vi "Experiment 6.vi"() -> ()   [LabVIEW 2026]
doc: "Experiment 6"
uses:
  <vilib>/Analysis/baseanly.llb/Mean (DBL).vi
  <vilib>/Analysis/NI_AALBase.lvlib
panel:
  out "Execution Time - Per Call (us)":dbl format="%.6f"
  out "Execution Time - 1M Calls (seconds)":dbl format="%.6f"
  out "Output":dbl[](array[numeric]) format="%.3f"
  # "Experiment 6"
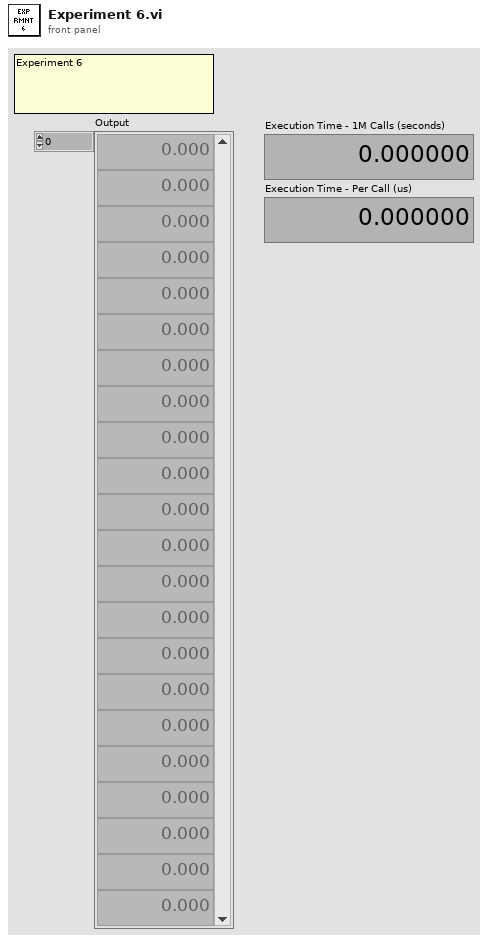
[diagram p1: front panel]
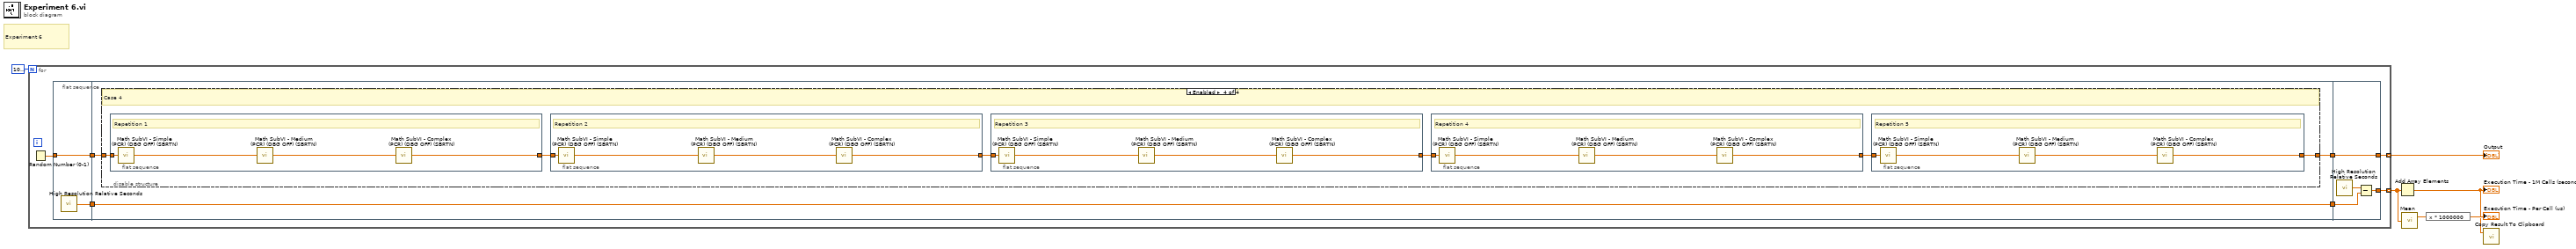
[diagram p0: block diagram]
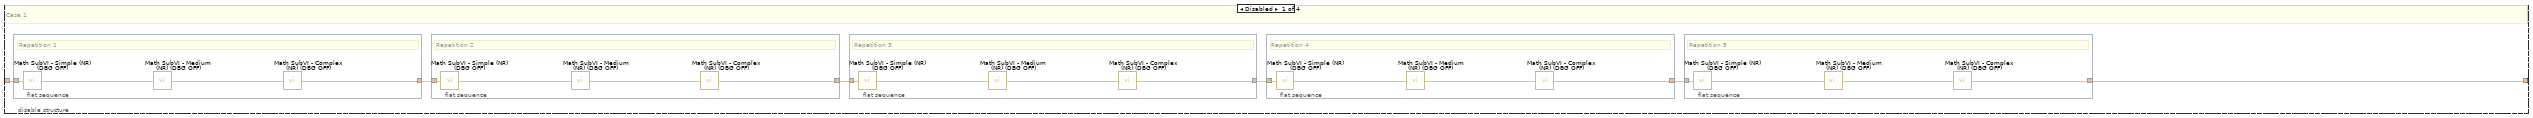
[diagram p2: hidden frame]
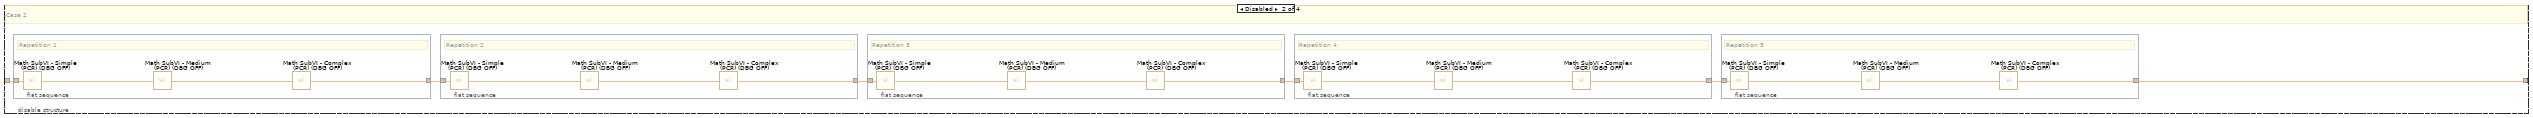
[diagram p3: hidden frame]
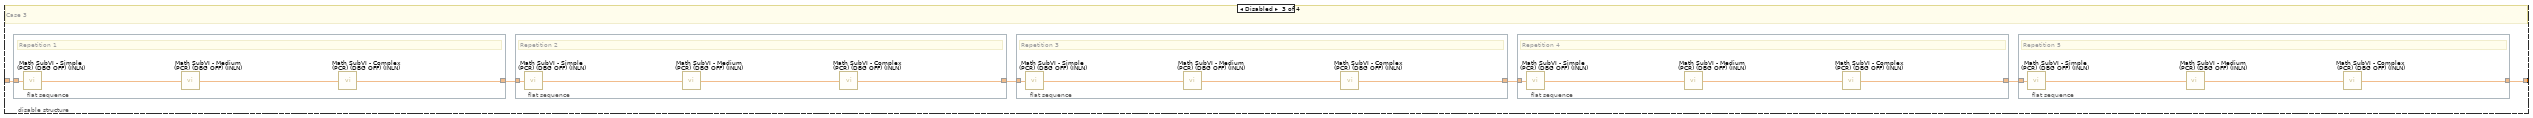
[diagram p4: hidden frame]
diagram:
  # "Experiment 6"
  n1 = for {
    N: 1000000 -> [_]
    tunnel: [w13] -> w6 mode=indexing
    tunnel: [w7] -> w4 mode=indexing
    n2 = Random Number (0-1)() -> (number: 0 to 1=w12:dbl)
    n3 = flat-sequence {
      tunnel: w12 -> [w15]
      tunnel: [w15] -> w11
      tunnel: [w14] -> w8
      tunnel: w11 -> [w16]
      tunnel: [w17] -> w10
      tunnel: [w18] -> w9
      tunnel: w8 -> [w18]
      tunnel: [w126] -> w13
      tunnel: w10 -> [w126]
      tunnel: w9 -> [w124]
      tunnel: [w123] -> w7
      frame #0 {
        n4 = call <vilib>:"High Resolution Relative Seconds.vi"() -> ("relative seconds"=w14:dbl)
      }
      frame #1 {
        n5 = disable-structure shown="Enabled" {
          disable-tunnel: [w19 w45 w71 w97] -> w17
          disable-tunnel: w16 -> [w24 w50 w76 w102]
          frame Disabled {
            # "Case 1"
            n6 = flat-sequence {
              tunnel: w24 -> [w43]
              tunnel: [w41] -> w23
              frame #0 {
                # "Repetition 1"
                n7 = call "Math SubVI - Simple (NR) (DBG OFF).vi"("Input"=w43) -> ("Output"=w44:dbl)
                n8 = call "Math SubVI - Medium (NR) (DBG OFF).vi"("Input"=w44) -> ("Output"=w42:dbl)
                n9 = call "Math SubVI - Complex (NR) (DBG OFF).vi"("Input"=w42) -> ("Output"=w41:dbl)
              }
            }
            n10 = flat-sequence {
              tunnel: w23 -> [w39]
              tunnel: [w37] -> w22
              frame #0 {
                # "Repetition 2"
                n11 = call "Math SubVI - Simple (NR) (DBG OFF).vi"("Input"=w39) -> ("Output"=w40:dbl)
                n12 = call "Math SubVI - Medium (NR) (DBG OFF).vi"("Input"=w40) -> ("Output"=w38:dbl)
                n13 = call "Math SubVI - Complex (NR) (DBG OFF).vi"("Input"=w38) -> ("Output"=w37:dbl)
              }
            }
            n14 = flat-sequence {
              tunnel: w22 -> [w35]
              tunnel: [w33] -> w21
              frame #0 {
                # "Repetition 3"
                n15 = call "Math SubVI - Simple (NR) (DBG OFF).vi"("Input"=w35) -> ("Output"=w36:dbl)
                n16 = call "Math SubVI - Medium (NR) (DBG OFF).vi"("Input"=w36) -> ("Output"=w34:dbl)
                n17 = call "Math SubVI - Complex (NR) (DBG OFF).vi"("Input"=w34) -> ("Output"=w33:dbl)
              }
            }
            n18 = flat-sequence {
              tunnel: w21 -> [w31]
              tunnel: [w29] -> w20
              frame #0 {
                # "Repetition 4"
                n19 = call "Math SubVI - Simple (NR) (DBG OFF).vi"("Input"=w31) -> ("Output"=w32:dbl)
                n20 = call "Math SubVI - Medium (NR) (DBG OFF).vi"("Input"=w32) -> ("Output"=w30:dbl)
                n21 = call "Math SubVI - Complex (NR) (DBG OFF).vi"("Input"=w30) -> ("Output"=w29:dbl)
              }
            }
            n22 = flat-sequence {
              tunnel: w20 -> [w27]
              tunnel: [w25] -> w19
              frame #0 {
                # "Repetition 5"
                n23 = call "Math SubVI - Simple (NR) (DBG OFF).vi"("Input"=w27) -> ("Output"=w28:dbl)
                n24 = call "Math SubVI - Medium (NR) (DBG OFF).vi"("Input"=w28) -> ("Output"=w26:dbl)
                n25 = call "Math SubVI - Complex (NR) (DBG OFF).vi"("Input"=w26) -> ("Output"=w25:dbl)
              }
            }
          }
          frame Disabled {
            # "Case 2"
            n26 = flat-sequence {
              tunnel: w50 -> [w69]
              tunnel: [w67] -> w49
              frame #0 {
                # "Repetition 1"
                n27 = call "Math SubVI - Simple (PCR) (DBG OFF).vi"("Input"=w69) -> ("Output"=w70:dbl)
                n28 = call "Math SubVI - Medium (PCR) (DBG OFF).vi"("Input"=w70) -> ("Output"=w68:dbl)
                n29 = call "Math SubVI - Complex (PCR) (DBG OFF).vi"("Input"=w68) -> ("Output"=w67:dbl)
              }
            }
            n30 = flat-sequence {
              tunnel: w49 -> [w65]
              tunnel: [w63] -> w48
              frame #0 {
                # "Repetition 2"
                n31 = call "Math SubVI - Simple (PCR) (DBG OFF).vi"("Input"=w65) -> ("Output"=w66:dbl)
                n32 = call "Math SubVI - Medium (PCR) (DBG OFF).vi"("Input"=w66) -> ("Output"=w64:dbl)
                n33 = call "Math SubVI - Complex (PCR) (DBG OFF).vi"("Input"=w64) -> ("Output"=w63:dbl)
              }
            }
            n34 = flat-sequence {
              tunnel: w48 -> [w61]
              tunnel: [w59] -> w47
              frame #0 {
                # "Repetition 3"
                n35 = call "Math SubVI - Simple (PCR) (DBG OFF).vi"("Input"=w61) -> ("Output"=w62:dbl)
                n36 = call "Math SubVI - Medium (PCR) (DBG OFF).vi"("Input"=w62) -> ("Output"=w60:dbl)
                n37 = call "Math SubVI - Complex (PCR) (DBG OFF).vi"("Input"=w60) -> ("Output"=w59:dbl)
              }
            }
            n38 = flat-sequence {
              tunnel: w47 -> [w57]
              tunnel: [w55] -> w46
              frame #0 {
                # "Repetition 4"
                n39 = call "Math SubVI - Simple (PCR) (DBG OFF).vi"("Input"=w57) -> ("Output"=w58:dbl)
                n40 = call "Math SubVI - Medium (PCR) (DBG OFF).vi"("Input"=w58) -> ("Output"=w56:dbl)
                n41 = call "Math SubVI - Complex (PCR) (DBG OFF).vi"("Input"=w56) -> ("Output"=w55:dbl)
              }
            }
            n42 = flat-sequence {
              tunnel: w46 -> [w53]
              tunnel: [w51] -> w45
              frame #0 {
                # "Repetition 5"
                n43 = call "Math SubVI - Simple (PCR) (DBG OFF).vi"("Input"=w53) -> ("Output"=w54:dbl)
                n44 = call "Math SubVI - Medium (PCR) (DBG OFF).vi"("Input"=w54) -> ("Output"=w52:dbl)
                n45 = call "Math SubVI - Complex (PCR) (DBG OFF).vi"("Input"=w52) -> ("Output"=w51:dbl)
              }
            }
          }
          frame Disabled {
            # "Case 3"
            n46 = flat-sequence {
              tunnel: w76 -> [w95]
              tunnel: [w93] -> w75
              frame #0 {
                # "Repetition 1"
                n47 = call "Math SubVI - Simple (PCR) (DBG OFF) (INLN).vi"("Input"=w95) -> ("Output"=w96:dbl)
                n48 = call "Math SubVI - Medium (PCR) (DBG OFF) (INLN).vi"("Input"=w96) -> ("Output"=w94:dbl)
                n49 = call "Math SubVI - Complex (PCR) (DBG OFF) (INLN).vi"("Input"=w94) -> ("Output"=w93:dbl)
              }
            }
            n50 = flat-sequence {
              tunnel: w75 -> [w91]
              tunnel: [w89] -> w74
              frame #0 {
                # "Repetition 2"
                n51 = call "Math SubVI - Simple (PCR) (DBG OFF) (INLN).vi"("Input"=w91) -> ("Output"=w92:dbl)
                n52 = call "Math SubVI - Medium (PCR) (DBG OFF) (INLN).vi"("Input"=w92) -> ("Output"=w90:dbl)
                n53 = call "Math SubVI - Complex (PCR) (DBG OFF) (INLN).vi"("Input"=w90) -> ("Output"=w89:dbl)
              }
            }
            n54 = flat-sequence {
              tunnel: w74 -> [w87]
              tunnel: [w85] -> w73
              frame #0 {
                # "Repetition 3"
                n55 = call "Math SubVI - Simple (PCR) (DBG OFF) (INLN).vi"("Input"=w87) -> ("Output"=w88:dbl)
                n56 = call "Math SubVI - Medium (PCR) (DBG OFF) (INLN).vi"("Input"=w88) -> ("Output"=w86:dbl)
                n57 = call "Math SubVI - Complex (PCR) (DBG OFF) (INLN).vi"("Input"=w86) -> ("Output"=w85:dbl)
              }
            }
            n58 = flat-sequence {
              tunnel: w73 -> [w83]
              tunnel: [w81] -> w72
              frame #0 {
                # "Repetition 4"
                n59 = call "Math SubVI - Simple (PCR) (DBG OFF) (INLN).vi"("Input"=w83) -> ("Output"=w84:dbl)
                n60 = call "Math SubVI - Medium (PCR) (DBG OFF) (INLN).vi"("Input"=w84) -> ("Output"=w82:dbl)
                n61 = call "Math SubVI - Complex (PCR) (DBG OFF) (INLN).vi"("Input"=w82) -> ("Output"=w81:dbl)
              }
            }
            n62 = flat-sequence {
              tunnel: w72 -> [w79]
              tunnel: [w77] -> w71
              frame #0 {
                # "Repetition 5"
                n63 = call "Math SubVI - Simple (PCR) (DBG OFF) (INLN).vi"("Input"=w79) -> ("Output"=w80:dbl)
                n64 = call "Math SubVI - Medium (PCR) (DBG OFF) (INLN).vi"("Input"=w80) -> ("Output"=w78:dbl)
                n65 = call "Math SubVI - Complex (PCR) (DBG OFF) (INLN).vi"("Input"=w78) -> ("Output"=w77:dbl)
              }
            }
          }
          frame Enabled {
            # "Case 4"
            n66 = flat-sequence {
              tunnel: w102 -> [w121]
              tunnel: [w119] -> w101
              frame #0 {
                # "Repetition 1"
                n67 = call "Math SubVI - Simple (PCR) (DBG OFF) (SBRTN).vi"("Input"=w121) -> ("Output"=w122:dbl)
                n68 = call "Math SubVI - Medium (PCR) (DBG OFF) (SBRTN).vi"("Input"=w122) -> ("Output"=w120:dbl)
                n69 = call "Math SubVI - Complex (PCR) (DBG OFF) (SBRTN).vi"("Input"=w120) -> ("Output"=w119:dbl)
              }
            }
            n70 = flat-sequence {
              tunnel: w101 -> [w117]
              tunnel: [w115] -> w100
              frame #0 {
                # "Repetition 2"
                n71 = call "Math SubVI - Simple (PCR) (DBG OFF) (SBRTN).vi"("Input"=w117) -> ("Output"=w118:dbl)
                n72 = call "Math SubVI - Medium (PCR) (DBG OFF) (SBRTN).vi"("Input"=w118) -> ("Output"=w116:dbl)
                n73 = call "Math SubVI - Complex (PCR) (DBG OFF) (SBRTN).vi"("Input"=w116) -> ("Output"=w115:dbl)
              }
            }
            n74 = flat-sequence {
              tunnel: w100 -> [w113]
              tunnel: [w111] -> w99
              frame #0 {
                # "Repetition 3"
                n75 = call "Math SubVI - Simple (PCR) (DBG OFF) (SBRTN).vi"("Input"=w113) -> ("Output"=w114:dbl)
                n76 = call "Math SubVI - Medium (PCR) (DBG OFF) (SBRTN).vi"("Input"=w114) -> ("Output"=w112:dbl)
                n77 = call "Math SubVI - Complex (PCR) (DBG OFF) (SBRTN).vi"("Input"=w112) -> ("Output"=w111:dbl)
              }
            }
            n78 = flat-sequence {
              tunnel: w99 -> [w109]
              tunnel: [w107] -> w98
              frame #0 {
                # "Repetition 4"
                n79 = call "Math SubVI - Simple (PCR) (DBG OFF) (SBRTN).vi"("Input"=w109) -> ("Output"=w110:dbl)
                n80 = call "Math SubVI - Medium (PCR) (DBG OFF) (SBRTN).vi"("Input"=w110) -> ("Output"=w108:dbl)
                n81 = call "Math SubVI - Complex (PCR) (DBG OFF) (SBRTN).vi"("Input"=w108) -> ("Output"=w107:dbl)
              }
            }
            n82 = flat-sequence {
              tunnel: w98 -> [w105]
              tunnel: [w103] -> w97
              frame #0 {
                # "Repetition 5"
                n83 = call "Math SubVI - Simple (PCR) (DBG OFF) (SBRTN).vi"("Input"=w105) -> ("Output"=w106:dbl)
                n84 = call "Math SubVI - Medium (PCR) (DBG OFF) (SBRTN).vi"("Input"=w106) -> ("Output"=w104:dbl)
                n85 = call "Math SubVI - Complex (PCR) (DBG OFF) (SBRTN).vi"("Input"=w104) -> ("Output"=w103:dbl)
              }
            }
          }
        }
      }
      frame #2 {
        n86 = call <vilib>:"High Resolution Relative Seconds.vi"() -> ("relative seconds"=w125:dbl)
        n87 = Subtract(x=w125, y=w124) -> (x-y=w123:dbl)
      }
    }
  }
  "Output" <- w6
  n88 = Add Array Elements(numeric array=w4) -> (sum=w1:dbl)
  "Execution Time - 1M Calls (seconds)" <- w1
  n89 = call-poly <vilib>:"Mean.vi"("X"=w4) -> ("mean"=w3:dbl)  [unwired: 1 out]
  n90 = expression code="x * 1000000"(w3) -> (→"Execution Time - Per Call (us)":dbl)
  n91 = call "Copy Result To Clipboard.vi"("Input"=w1) -> ()  [unwired: 1 in]
